vi "ZM_state.vi"(6 "ZB01":bool, 9 "Z_State":T1, 10 "Z_Source (hand)":T2=enum."hand", 11 "ZM_state in":refnum<class "valve_VCH_ZM_state.lvclass">) -> (3 "ZM_state out":refnum<class "valve_VCH_ZM_state.lvclass">)   [LabVIEW 2019, in "valve_VCH_ZM_state.lvclass"]
uses:
  valve_VCH_ZM_state.lvclass
  D:/my_projects/projects/Algorithms/Labview/19/Sequence/State/State.lvclass
  Heating/ctl/Z_source.ctl
  ctl/Z_State_VCH.ctl
  ctl/ZM_State_VCH.ctl
  valve_VCH_ZM_state.lvclass/valve_VCH_ZM_state.ctl
  Valves.lvlib
  Sequence/State/State.lvclass
  Heating/Heating.lvlib
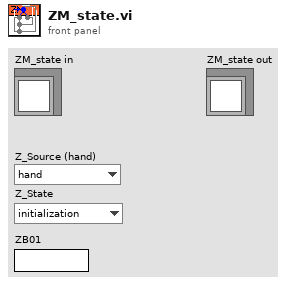
[diagram p1: front panel]
types:
  T1 = typedef "Valves.lvlib/Z_State_VCH.ctl" = enum8{"initialization", "alarm", "disabled", "not ready", "closed ready", "reserv", "reserv1", "reserv2", "reserv3", "check", "on min", "open", "on (closed)"}
  T2 = typedef "Heating.lvlib/Z_source.ctl" = enum8{"initialize", "local disabled", "local hand", "hand", "auto", "dist"}
  T3 = typedef "Valves.lvlib/ZM_State_VCH.ctl" = enum8{"initialization", "closed", "big_pause", "little_pause", "open", "close_cmd"}
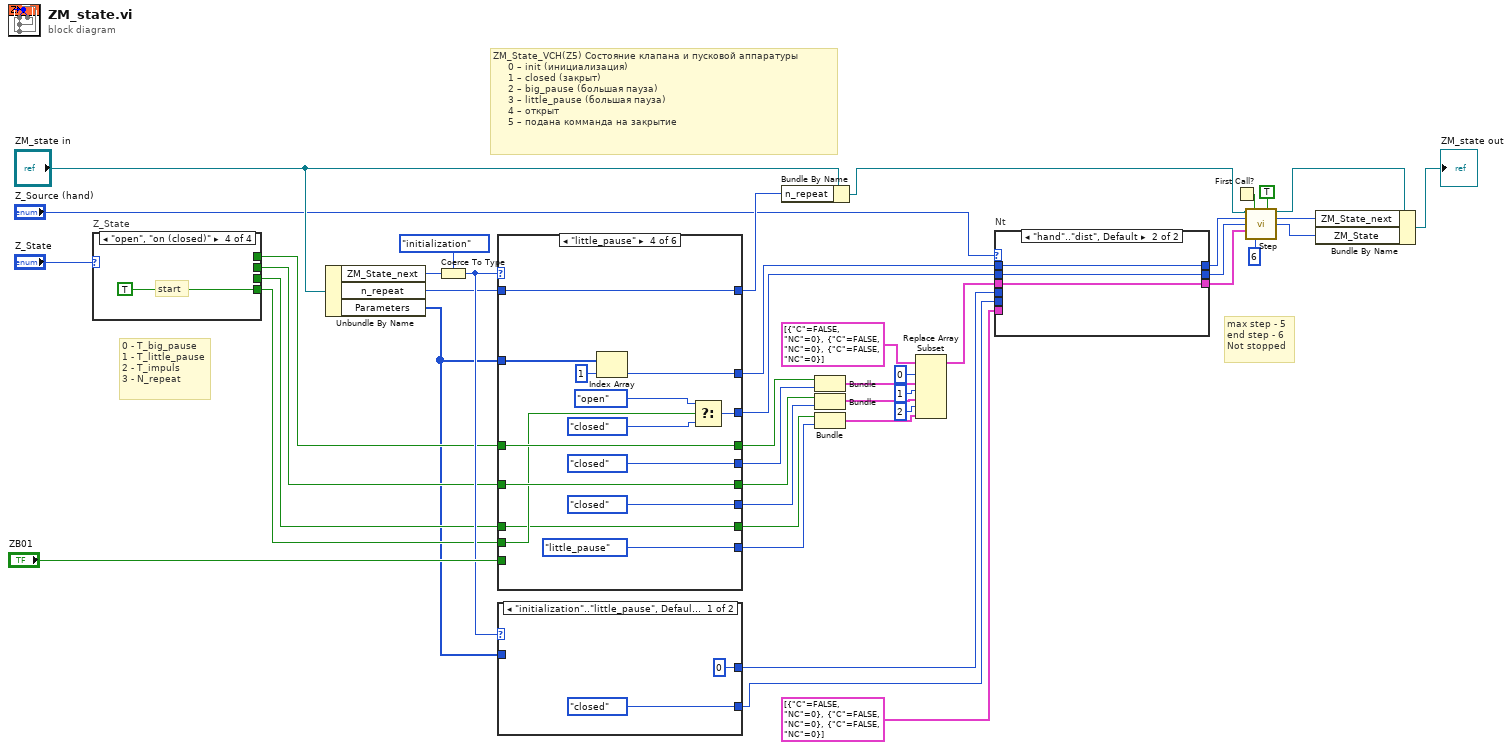
[diagram p0: block diagram]
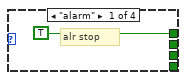
[diagram p2: hidden frame]
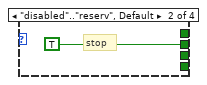
[diagram p3: hidden frame]
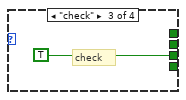
[diagram p4: hidden frame]
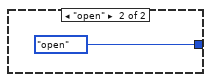
[diagram p6: hidden frame]
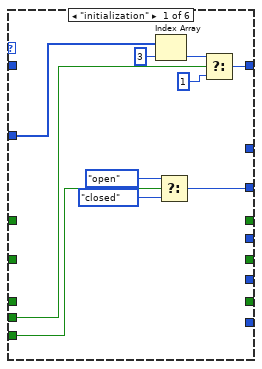
[diagram p7: hidden frame]
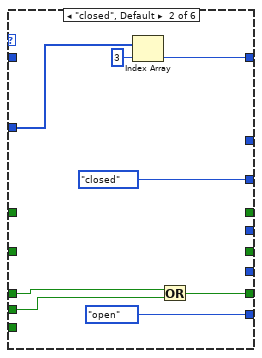
[diagram p8: hidden frame]
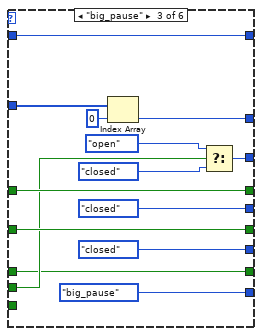
[diagram p9: hidden frame]
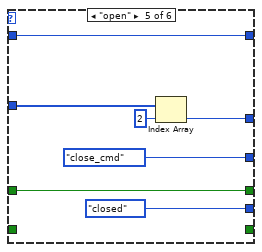
[diagram p10: hidden frame]
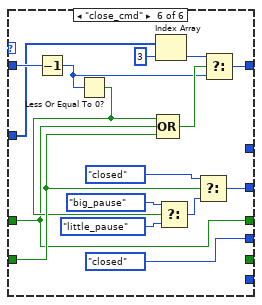
[diagram p11: hidden frame]
diagram:
  # "ZM_State_VCH(Z5) Состояние клапана и пусковой аппаратуры\n     0 – init (инициализация)\n     1 – сlosed (закрыт)\n     2 – big_pause (большая пауза)\n     3 – little_pause (большая пауза)\n     4 – открыт\n     5 – подана комманда на закрытие"
  # "max step - 5\nend step - 6\nNot stopped"
  # "0 - T_big_pause\n1 - T_little_pause\n2 - T_impuls\n3 - N_repeat"
  n1 = case "Z_State" shown="\"open\", \"on (closed)\"" "Z_State" {
    tunnel: [_ TRUE _ _] -> w25
    tunnel: [_ _ TRUE _] -> w24
    tunnel: [TRUE _ _ _] -> w26
    tunnel: [_ _ _ TRUE] -> w23
    frame "alarm" {
      # "alr stop"
    }
    frame "disabled".."reserv", Default {
      # "stop"
    }
    frame "check" {
      # "check"
    }
    frame "open", "on (closed)" {
      # "start"
    }
  }
  n2 = Unbundle By Name("ZM_state in") -> ("ZM_State_next"=w8:T3, "n_repeat"=w10:u32, "Parameters"=w7:u32[])
  n3 = Coerce To Type(0:w8, 1:ZM_State_VCH."initialization" ("ZM_State_VCH")) -> (2:w42:T3)
  n4 = case shown="\"little_pause\"" w42 {
    tunnel: w7 -> [w57 w60 w79 w93 w99 w113]
    tunnel: [w56 ZM_State_VCH."closed" ("ZM_State_VCH") w75 w89 ZM_State_VCH."close_cmd" ("ZM_State_VCH") w109] -> w22
    tunnel: [_ _ w69 w83 w100 _] -> w19
    tunnel: [_ _ w77 w91 w97 w102] -> w28
    tunnel: [_ _ ZM_State_VCH."closed" ("ZM_State_VCH") ZM_State_VCH."closed" ("ZM_State_VCH") ZM_State_VCH."closed" ("ZM_State_VCH") ZM_State_VCH."closed" ("ZM_State_VCH")] -> w29
    tunnel: [_ w65 w68 w82 _ _] -> w32
    tunnel: w24 -> [_ w66 w68 w82 _ _]
    tunnel: [_ ZM_State_VCH."open" ("ZM_State_VCH") ZM_State_VCH."big_pause" ("ZM_State_VCH") ZM_State_VCH."little_pause" ("ZM_State_VCH") _ _] -> w33
    tunnel: w25 -> [_ _ w76 w90 _ w108]
    tunnel: [_ _ w76 w90 _ _] -> w30
    tunnel: [_ _ ZM_State_VCH."closed" ("ZM_State_VCH") ZM_State_VCH."closed" ("ZM_State_VCH") _ _] -> w31
    tunnel: w26 -> [_ _ w77 w91 w97 w102]
    tunnel: "ZB01" -> [w55 _ _ _ _ _]
    tunnel: [w54 w59 w78 w92 w96 w114] -> w11
    tunnel: w10 -> [_ _ w78 w92 w96 w115]
    tunnel: w23 -> [w51 w64 w74 w88 _ _]
    frame "initialization" {
      n5 = Index Array(array=w57, index=3) -> (element=w53:u32)
      n6 = Select(t=ZM_State_VCH."open" ("ZM_State_VCH"), s=w55, f=ZM_State_VCH."closed" ("ZM_State_VCH")) -> (s? t:f=w56:T3)
      n7 = Select(t=w53, s=w51, f=u32 1 ("End step")) -> (s? t:f=w54:u32)
    }
    frame "closed", Default {
      n8 = Index Array(array=w60, index=3) -> (element=w59:u32)
      n9 = Or(x=w66, y=w64) -> (x .or. y?=w65:bool)
    }
    frame "big_pause" {
      n10 = Index Array(array=w79, index=0) -> (element=w69:u32)
      n11 = Select(t=ZM_State_VCH."open" ("ZM_State_VCH"), s=w74, f=ZM_State_VCH."closed" ("ZM_State_VCH")) -> (s? t:f=w75:T3)
    }
    frame "little_pause" {
      n12 = Index Array(array=w93, index=1) -> (element=w83:u32)
      n13 = Select(t=ZM_State_VCH."open" ("ZM_State_VCH"), s=w88, f=ZM_State_VCH."closed" ("ZM_State_VCH")) -> (s? t:f=w89:T3)
    }
    frame "open" {
      n14 = Index Array(array=w99, index=2) -> (element=w100:u32)
    }
    frame "close_cmd" {
      n15 = Decrement(x=w115) -> (x-1=w111:u32)
      n16 = Less Or Equal To 0?(x=w111) -> (x <= 0?=w103:bool)
      n17 = Index Array(array=w113, index=3) -> (element=w117:u32)
      n18 = Compound Arithmetic op=OR(w103, w102, w108) -> (w112:bool)
      n19 = Select(t=ZM_State_VCH."big_pause" ("ZM_State_VCH"), s=w103, f=ZM_State_VCH."little_pause" ("ZM_State_VCH")) -> (s? t:f=w110:T3)
      n20 = Select(t=ZM_State_VCH."closed" ("ZM_State_VCH"), s=w108, f=w110) -> (s? t:f=w109:T3)
      n21 = Select(t=w117, s=w112, f=w111) -> (s? t:f=w114:u32)
    }
  }
  n22 = case shown="\"initialization\"..\"little_pause\", Default" w42 {
    tunnel: w7 -> [_ _]
    tunnel: [ZM_State_VCH."closed" ("ZM_State_VCH") ZM_State_VCH."open" ("ZM_State_VCH")] -> w21
    tunnel: [u32 0 ("pump param") _] -> w20
    frame "initialization".."little_pause", Default {
    }
    frame "open" {
    }
  }
  n23 = Bundle By Name(cluster="ZM_state in", "n_repeat"=w11) -> (w2:refnum<class "valve_VCH_ZM_state.lvclass">)
  n24 = Bundle(w28, "ZM_State_VCH"=w29) -> (w39:cluster{bool, "ZM_State_VCH":T3})  [unwired: 1 in]
  n25 = Bundle(w30, "ZM_State_VCH"=w31) -> (w36:cluster{bool, "ZM_State_VCH":T3})  [unwired: 1 in]
  n26 = Bundle(w32, "ZM_State_VCH"=w33) -> (w35:cluster{bool, "ZM_State_VCH":T3})  [unwired: 1 in]
  n27 = Replace Array Subset(array=cluster{"C":bool, "NC":u32}[] [{"C"=FALSE, "NC"=0}, {"C"=FALSE, "NC"=0}, {"C"=FALSE, "NC"=0}] ("appended array"), new element #1=w39, index #1=0 ("index"), new element #2=w36, index #2=1 ("index"), new element #3=w35, index #3=2 ("index")) -> (w34:cluster{"C":bool, "NC":u32}[])
  n28 = case "Nt" shown="\"hand\"..\"dist\", Default" "Z_Source (hand)" {
    tunnel: w22 -> [_ w126]
    tunnel: w34 -> [_ w125]
    tunnel: [w122 w126] -> w16
    tunnel: [w123 w125] -> w15
    tunnel: w21 -> [w122 _]
    tunnel: cluster{"C":bool, "NC":u32}[] [{"C"=FALSE, "NC"=0}, {"C"=FALSE, "NC"=0}, {"C"=FALSE, "NC"=0}] ("appended array") -> [w123 _]
    tunnel: w20 -> [w121 _]
    tunnel: [w121 w124] -> w17
    tunnel: w19 -> [_ w124]
    frame "local disabled", "local hand" {
    }
    frame "hand".."dist", Default {
    }
  }
  n29 = First Call?() -> (First Call?: T/F=w18:bool)
  n30 = call "Step.vi"("State in"=w2, "Reset"=w18, "Start in"=TRUE ("Start"), "t"=w17, "Nt"=w16, "C_table"=w15, "N end step"=u32 6) -> ("State out"=w1:refnum<class "valve_VCH_ZM_state.lvclass">, "N next"=w12:u32, "N curr"=w13:u32)  [unwired: 5 in, 1 out]
  n31 = Bundle By Name(cluster=w1, "ZM_State_next"=w12, "ZM_State"=w13) -> (→"ZM_state out":refnum<class "valve_VCH_ZM_state.lvclass">)
